vi "FTW-Scheduler-Construct.vi"(1 "Initial Job Sequence":string) -> (0 "FTW Job Scheduler":refnum<class "FTW-Scheduler.lvclass">)   [LabVIEW 2013, in "FTW-Scheduler.lvclass"]
uses:
  FTW-Scheduler.lvclass
  FTW-Scheduler.lvclass/FTW-Scheduler.ctl
panel:
  # "Inputs"
  # "Outputs"
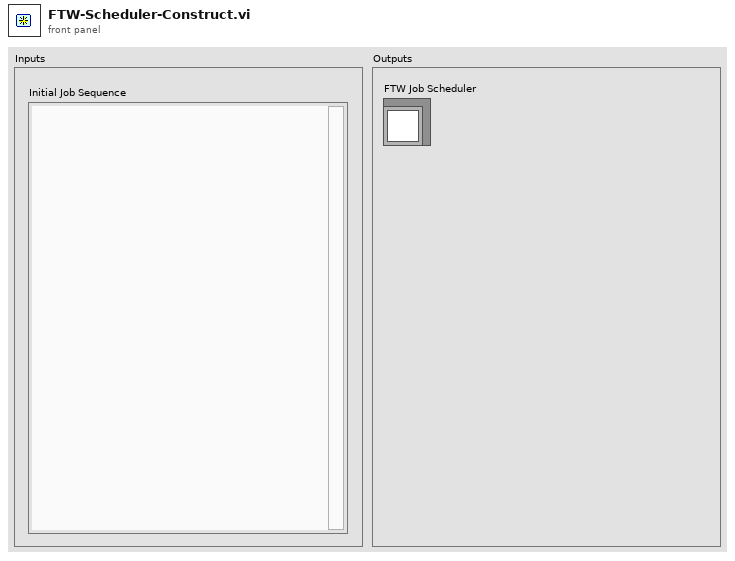
[diagram p1: front panel]
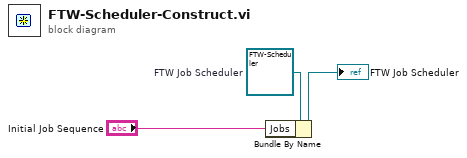
[diagram p0: block diagram]
diagram:
  w3 = refnum<class "FTW-Scheduler.lvclass"> refnum  # FTW Job Scheduler
  n1 = Bundle By Name(cluster=w3, "Jobs"="Initial Job Sequence") -> (→"FTW Job Scheduler":refnum<class "FTW-Scheduler.lvclass">)
